vi "Export File - Rx Packet XML.vi"(4 "Rx Packet":T2 {"Endianness" items=["big-endian"=0, "little-endian"=2]}, 6 "RootNode":refnum<k24>, 8 "error in (no error)":errorcluster, 9 "Rx Packet Header Data":T1, 11 "XmlDocument in":refnum<k24>) -> (0 "error out":errorcluster, 3 "XmlDocument out":refnum<k24>)   [LabVIEW 2016, in "UDP-Custom-Device System Explorer.lvlib"]
uses:
  UDP-Custom-Device System Explorer.lvlib
  System.Xml
  Types/XML - New/ImpExp - Rx Packet Data.ctl
  <vilib>/NI Veristand/Custom Device API/Custom Device Item Info.ctl
  Shared/Types/Shared - Channel Data Type.ctl
  Shared/Types/Shared - Buffered.PacketInfo.ctl
  Shared/Types/Shared - Pointer Encoding.ctl
  Shared/Types/Shared - New Data Options.ctl
  Types/XML - New/ImpExp - Packet Headers.ctl
  Shared/UDP-Custom-Device Shared.lvlib
  <vilib>/NI VeriStand/Custom Device API/Custom Device API.lvlib
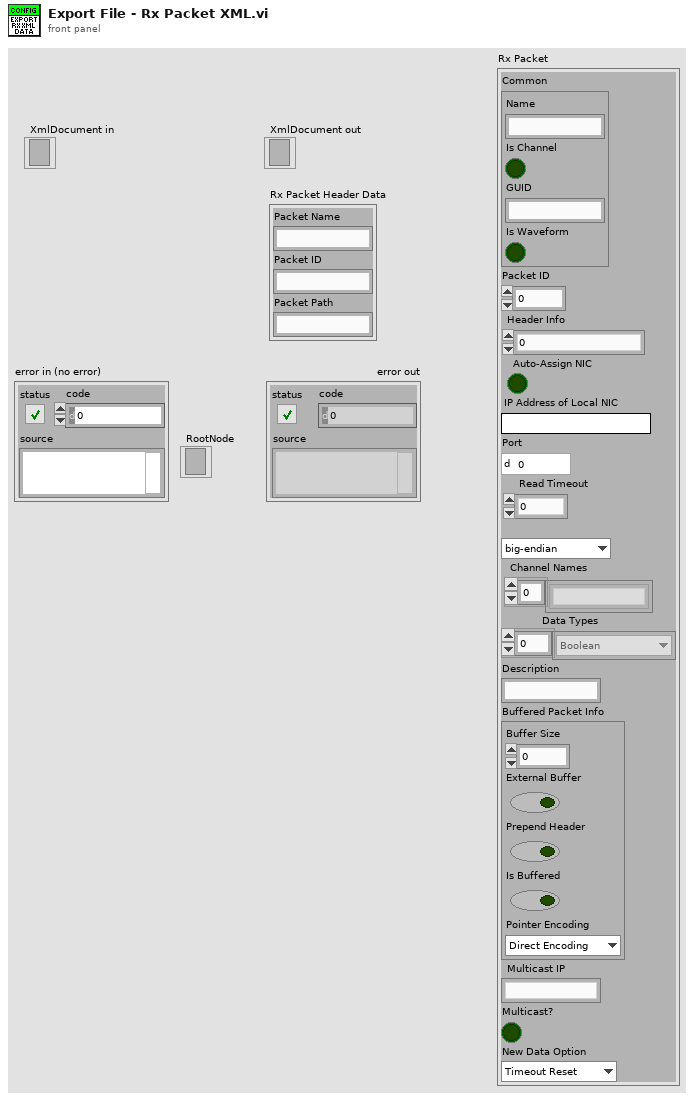
[diagram p1: front panel]
types:
  T1 = typedef "UDP-Custom-Device System Explorer.lvlib/ImpExp - Packet Headers.ctl" = cluster{"Packet Name":string, "Packet ID":string, "Packet Path":string}
  T2 = typedef "UDP-Custom-Device System Explorer.lvlib/ImpExp - Rx Packet Data.ctl" = cluster{"Common":T3, "Packet ID":i32, "Header Info":u32, "Auto-Assign NIC":bool, "IP Address of Local NIC":string, "Port":u16, "Read Timeout":i32, "Endianness":u16, "Channel Names":string[], "Data Types":T4[], "Description":string, "Buffered Packet Info":T5, "Multicast IP":string, "Multicast?":bool, "New Data Option":T7}
  T3 = typedef "Custom Device API.lvlib/Custom Device Item Info.ctl" = cluster{"Name":string, "Is Channel":bool, "GUID":string, "Is Waveform":bool}
  T4 = typedef "UDP-Custom-Device Shared.lvlib/Shared - Channel Data Type.ctl" = enum16{"Boolean", "Single", "Double", "I8", "I16", "I32", "I64", "U8", "U16", "U32", "U64"}
  T5 = typedef "UDP-Custom-Device Shared.lvlib/Shared - Buffered.PacketInfo.ctl" = cluster{"Buffer Size":i32, "External Buffer":bool, "Prepend Header":bool, "Is Buffered":bool, "Pointer Encoding":T6}
  T6 = typedef "UDP-Custom-Device Shared.lvlib/Shared - Pointer Encoding.ctl" = enum16{"Direct Encoding", "Conversion Encoding"}
  T7 = typedef "UDP-Custom-Device Shared.lvlib/Shared - New Data Options.ctl" = enum16{"Timeout Reset", "Counter"}
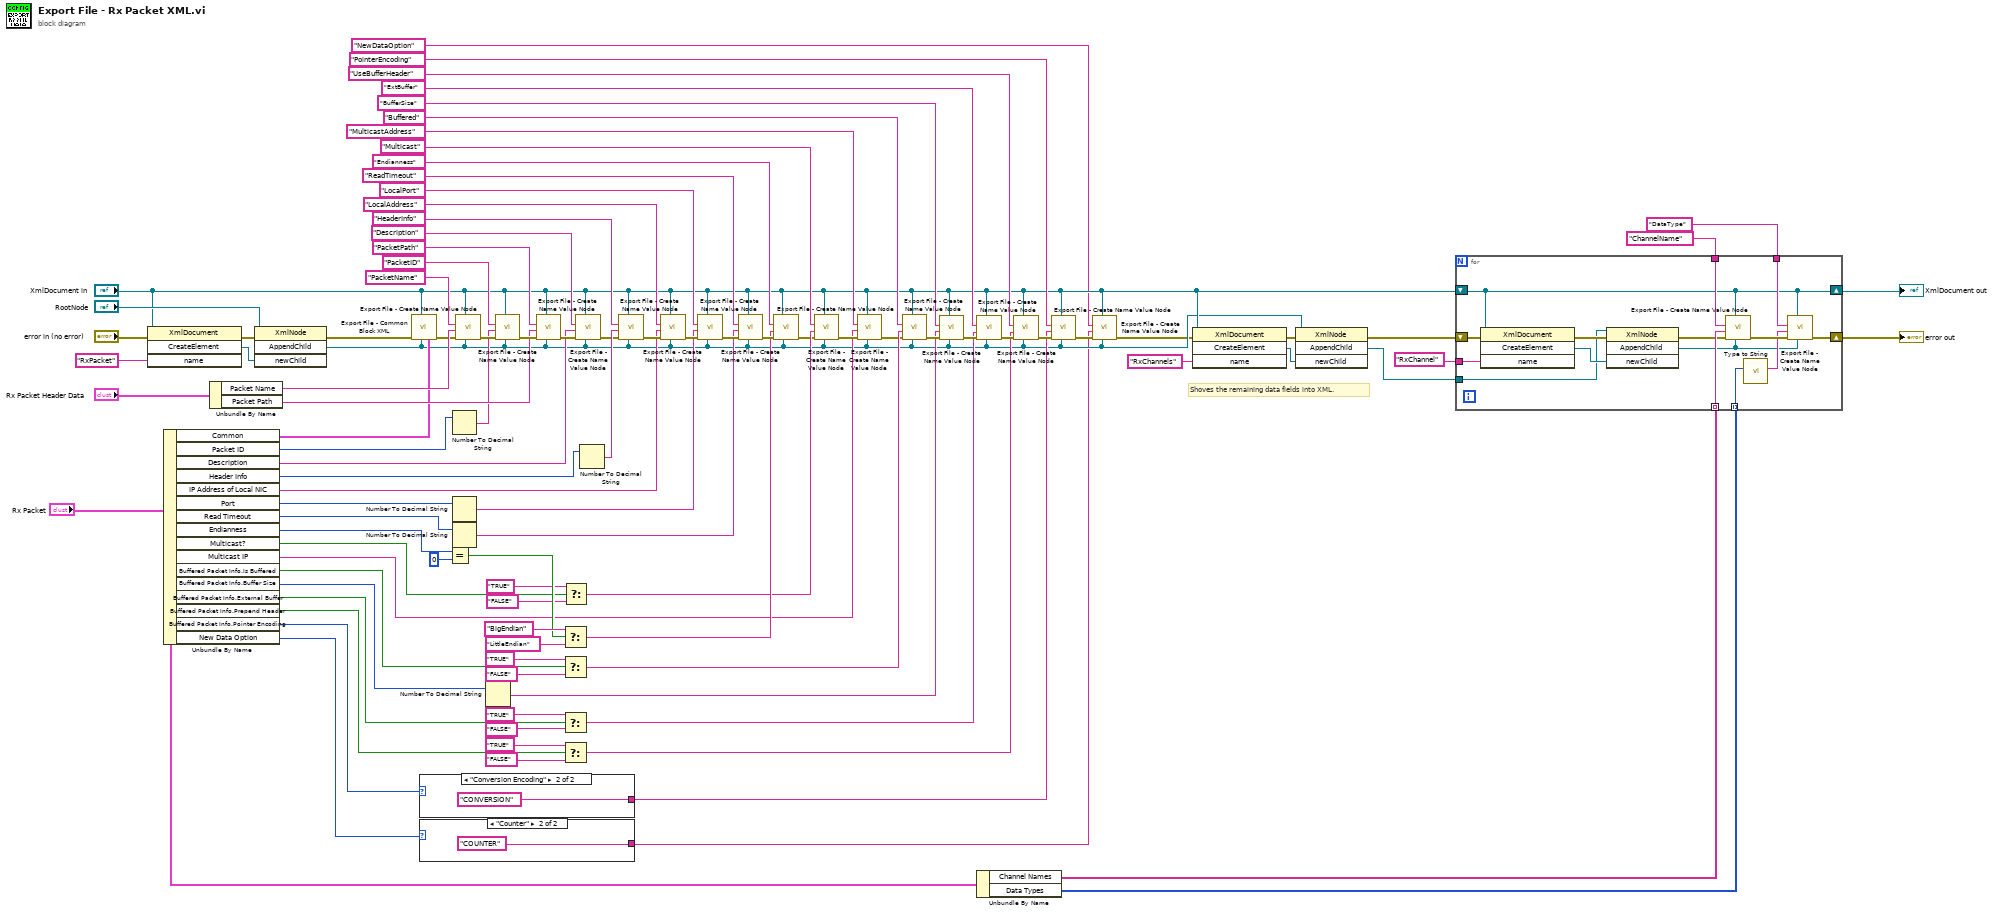
[diagram p0: block diagram]
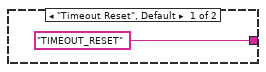
[diagram p2: hidden frame]
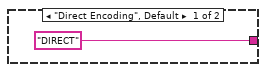
[diagram p3: hidden frame]
diagram:
  # "Shoves the remaining data fields into XML."
  n1 = invoke class="XmlDocument" method="CreateElement"(reference="XmlDocument in", error in="error in (no error)", "name"="RxPacket" ("Tag Name")) -> (error out=w89:errorcluster, "CreateElement"=w90:refnum<k24>)  [unwired: 1 in, 2 out]
  n2 = Unbundle By Name("Rx Packet") -> ("Common"=w84:T3, "Packet ID"=w59:i32, "Description"=w61:string, "Header Info"=w60:u32, "IP Address of Local NIC"=w73:string, "Port"=w71:u16, "Read Timeout"=w68:i32, "Endianness"=w66:u16, "Multicast?"=w19:bool, "Multicast IP"=w13:string, "Buffered Packet Info.Is Buffered"=w45:bool, "Buffered Packet Info.Buffer Size"=w46:i32, "Buffered Packet Info.External Buffer"=w44:bool, "Buffered Packet Info.Prepend Header"=w43:bool, "Buffered Packet Info.Pointer Encoding"=w11:T6, "New Data Option"=w2:T7)
  n3 = Unbundle By Name("Rx Packet Header Data") -> ("Packet Name"=w93:string, "Packet Path"=w92:string)
  n4 = invoke class="XmlNode" method="AppendChild"(reference="RootNode", error in=w89, "newChild"=w90) -> (error out=w85:errorcluster, "AppendChild"=w6:refnum<k24>)  [unwired: 1 in, 2 out]
  n5 = call "Export File - Common Block XML.vi"("Common"=w84, "RootNode in"=w6, "XmlDocument in"="XmlDocument in", "error in (no error)"=w85) -> ("error out"=w88:errorcluster)  [unwired: 7 in]
  n6 = case shown="\"Conversion Encoding\"" w11 {
    tunnel: ["DIRECT" "CONVERSION"] -> w8
    frame "Direct Encoding", Default {
    }
    frame "Conversion Encoding" {
    }
  }
  n7 = case shown="\"Counter\"" w2 {
    tunnel: ["TIMEOUT_RESET" "COUNTER"] -> w1
    frame "Timeout Reset", Default {
    }
    frame "Counter" {
    }
  }
  n8 = Equal?(x=w66, y=u16 0) -> (x = y?=w55:bool)
  n9 = Number To Decimal String(number=w59) -> (decimal integer string=w58:string)  [unwired: 1 in]
  n10 = Number To Decimal String(number=w71) -> (decimal integer string=w70:string)  [unwired: 1 in]
  n11 = Number To Decimal String(number=w68) -> (decimal integer string=w67:string)  [unwired: 1 in]
  n12 = call "Export File - Create Name Value Node.vi"("RootNode in"=w6, "XmlDocument in"="XmlDocument in", "error in (no error)"=w88, "Value"=w93, "Name"="PacketName" ("Tag Name")) -> ("error out"=w99:errorcluster)  [unwired: 6 in]
  n13 = Number To Decimal String(number=w46) -> (decimal integer string=w37:string)  [unwired: 1 in]
  n14 = call "Export File - Create Name Value Node.vi"("RootNode in"=w6, "XmlDocument in"="XmlDocument in", "error in (no error)"=w99, "Value"=w58, "Name"="PacketID" ("Tag Name")) -> ("error out"=w98:errorcluster)  [unwired: 6 in]
  n15 = call "Export File - Create Name Value Node.vi"("RootNode in"=w6, "XmlDocument in"="XmlDocument in", "error in (no error)"=w98, "Value"=w92, "Name"="PacketPath" ("Tag Name")) -> ("error out"=w64:errorcluster)  [unwired: 6 in]
  n16 = Select(t="BigEndian", s=w55, f="LittleEndian") -> (s? t:f=w54:string)
  n17 = Select(t="TRUE", s=w45, f="FALSE") -> (s? t:f=w38:string)
  n18 = Select(t="TRUE", s=w44, f="FALSE") -> (s? t:f=w36:string)
  n19 = Select(t="TRUE", s=w43, f="FALSE") -> (s? t:f=w35:string)
  n20 = Select(t="TRUE", s=w19, f="FALSE") -> (s? t:f=w14:string)
  n21 = call "Export File - Create Name Value Node.vi"("RootNode in"=w6, "XmlDocument in"="XmlDocument in", "error in (no error)"=w64, "Value"=w61, "Name"="Description" ("Tag Name")) -> ("error out"=w63:errorcluster)  [unwired: 6 in]
  n22 = Number To Decimal String(number=w60) -> (decimal integer string=w76:string)  [unwired: 1 in]
  n23 = call "Export File - Create Name Value Node.vi"("RootNode in"=w6, "XmlDocument in"="XmlDocument in", "error in (no error)"=w63, "Value"=w76, "Name"="HeaderInfo" ("Tag Name")) -> ("error out"=w83:errorcluster)  [unwired: 6 in]
  n24 = call "Export File - Create Name Value Node.vi"("RootNode in"=w6, "XmlDocument in"="XmlDocument in", "error in (no error)"=w83, "Value"=w73, "Name"="LocalAddress" ("Tag Name")) -> ("error out"=w82:errorcluster)  [unwired: 6 in]
  n25 = call "Export File - Create Name Value Node.vi"("RootNode in"=w6, "XmlDocument in"="XmlDocument in", "error in (no error)"=w82, "Value"=w70, "Name"="LocalPort" ("Tag Name")) -> ("error out"=w81:errorcluster)  [unwired: 6 in]
  n26 = call "Export File - Create Name Value Node.vi"("RootNode in"=w6, "XmlDocument in"="XmlDocument in", "error in (no error)"=w81, "Value"=w67, "Name"="ReadTimeout" ("Tag Name")) -> ("error out"=w80:errorcluster)  [unwired: 6 in]
  n27 = call "Export File - Create Name Value Node.vi"("RootNode in"=w6, "XmlDocument in"="XmlDocument in", "error in (no error)"=w80, "Value"=w54, "Name"="Endianness" ("Tag Name")) -> ("error out"=w12:errorcluster)  [unwired: 6 in]
  n28 = call "Export File - Create Name Value Node.vi"("RootNode in"=w6, "XmlDocument in"="XmlDocument in", "error in (no error)"=w12, "Value"=w14, "Name"="Multicast" ("Tag Name")) -> ("error out"=w18:errorcluster)  [unwired: 6 in]
  n29 = call "Export File - Create Name Value Node.vi"("RootNode in"=w6, "XmlDocument in"="XmlDocument in", "error in (no error)"=w18, "Value"=w13, "Name"="MulticastAddress" ("Tag Name")) -> ("error out"=w17:errorcluster)  [unwired: 6 in]
  n30 = call "Export File - Create Name Value Node.vi"("RootNode in"=w6, "XmlDocument in"="XmlDocument in", "error in (no error)"=w17, "Value"=w38, "Name"="Buffered" ("Tag Name")) -> ("error out"=w79:errorcluster)  [unwired: 6 in]
  n31 = call "Export File - Create Name Value Node.vi"("RootNode in"=w6, "XmlDocument in"="XmlDocument in", "error in (no error)"=w79, "Value"=w37, "Name"="BufferSize" ("Tag Name")) -> ("error out"=w78:errorcluster)  [unwired: 6 in]
  n32 = call "Export File - Create Name Value Node.vi"("RootNode in"=w6, "XmlDocument in"="XmlDocument in", "error in (no error)"=w78, "Value"=w36, "Name"="ExtBuffer" ("Tag Name")) -> ("error out"=w77:errorcluster)  [unwired: 6 in]
  n33 = Unbundle By Name("Rx Packet") -> ("Channel Names"=w24:string[], "Data Types"=w23:T4[])
  n34 = call "Export File - Create Name Value Node.vi"("RootNode in"=w6, "XmlDocument in"="XmlDocument in", "error in (no error)"=w77, "Value"=w35, "Name"="UseBufferHeader" ("Tag Name")) -> ("error out"=w10:errorcluster)  [unwired: 6 in]
  n35 = call "Export File - Create Name Value Node.vi"("RootNode in"=w6, "XmlDocument in"="XmlDocument in", "error in (no error)"=w10, "Value"=w8, "Name"="PointerEncoding" ("Tag Name")) -> ("error out"=w5:errorcluster)  [unwired: 6 in]
  n36 = call "Export File - Create Name Value Node.vi"("RootNode in"=w6, "XmlDocument in"="XmlDocument in", "error in (no error)"=w5, "Value"=w1, "Name"="NewDataOption" ("Tag Name")) -> ("error out"=w4:errorcluster)  [unwired: 6 in]
  n37 = invoke class="XmlDocument" method="CreateElement"(reference="XmlDocument in", error in=w4, "name"="RxChannels" ("Tag Name")) -> (error out=w31:errorcluster, "CreateElement"=w33:refnum<k24>)  [unwired: 1 in, 2 out]
  n38 = invoke class="XmlNode" method="AppendChild"(reference=w6, error in=w31, "newChild"=w33) -> (error out=w30:errorcluster, "AppendChild"=w28:refnum<k24>)  [unwired: 1 in, 2 out]
  n39 = for {
    shift-right: [w117] -> w29
    shift-left: w30 -> [w109]
    tunnel: w28 -> [w106]
    shift-right: [w110] -> w27
    shift-left: "XmlDocument in" -> [w110]
    tunnel: "ChannelName" ("Tag Name") -> [w116]
    tunnel: "DataType" ("Tag Name") -> [w115]
    tunnel: w24 -> [w114] mode=indexing
    tunnel: w23 -> [w113] mode=indexing
    tunnel: "RxChannel" ("Tag Name") -> [w107]
    n40 = invoke class="XmlDocument" method="CreateElement"(reference=w110, error in=w109, "name"=w107) -> (error out=w108:errorcluster, "CreateElement"=w111:refnum<k24>)  [unwired: 1 in, 2 out]
    n41 = invoke class="XmlNode" method="AppendChild"(reference=w106, error in=w108, "newChild"=w111) -> (error out=w104:errorcluster, "AppendChild"=w105:refnum<k24>)  [unwired: 1 in, 2 out]
    n42 = call "Export File - Create Name Value Node.vi"("RootNode in"=w105, "XmlDocument in"=w110, "error in (no error)"=w104, "Value"=w114, "Name"=w116) -> ("error out"=w118:errorcluster)  [unwired: 6 in]
    n43 = call "Type to String.vi"("Data Type"=w113) -> ("String Type"=w112:string)  [unwired: 10 in]
    n44 = call "Export File - Create Name Value Node.vi"("RootNode in"=w105, "XmlDocument in"=w110, "error in (no error)"=w118, "Value"=w112, "Name"=w115) -> ("error out"=w117:errorcluster)  [unwired: 6 in]
  }
  "error out" <- w29
  "XmlDocument out" <- w27
